vi "PPMS.TestLauncher.vi"() -> ()   [LabVIEW 2019, in "instrument.PPMS.lvclass"]
uses:
  instrument.PPMS.lvclass
  <vilib>/JKI/JKI SMO/SMO/SMO.lvclass
  <vilib>/JKI/JKI SMO/SMO/Typedefs/SMOState --Enum.ctl
  C:/Program Files (x86)/National Instruments/LabVIEW 2019/user.lib/LevyLab/Instrument Framework/Instrument Types/Cryostat/Instrument.Cryostat.lvclass
  C:/Program Files (x86)/National Instruments/LabVIEW 2019/user.lib/LevyLab/Instrument Framework/Instrument/Instrument.lvclass
  C:/Program Files (x86)/National Instruments/LabVIEW 2019/vi.lib/JKI/JKI SMO/SMO/SMO.lvclass
  <userlib>/LevyLab/Instrument Framework/Instrument/Instrument.lvclass
panel:
  in  "Debug Mode? [F]":bool
  out "SMO State":T1
  out "error out":errorcluster
  in  "Stop":bool
  # "PPMS Test Launcher"
  # "For instructions on how to use the JKI State Machine Objects, examples and video tutorials, visit:\nhttp://jki.net/state-machine-objects/\n\nJKI State Machine Objects™\nhttp://jki.net/state-machine-objects/\nCopyright (C) 2005-2015, JKI <info@jki.net>\nALL RIGHTS RESERVED"
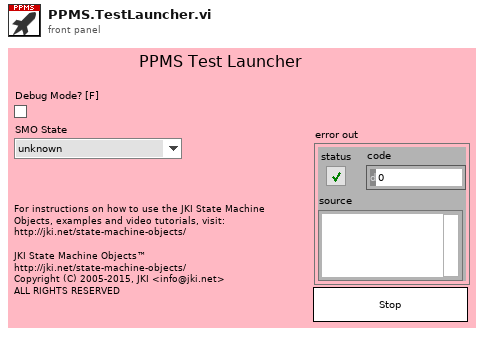
[diagram p1: front panel]
types:
  T1 = typedef "smo.lvlib/SMO.lvclass/SMOState --Enum.ctl" = enum16{"unknown", "Created", "Started", "Stopped"}
  T2 = typedef "smo.lvlib/SMO.lvclass/Public Events.ctl" = cluster{"Error":refnum<user-event>, "State":refnum<user-event>, "Reserve State":refnum<user-event>}
  T3 = cluster{"Event Registration Refnum":refnum<event-registration>}
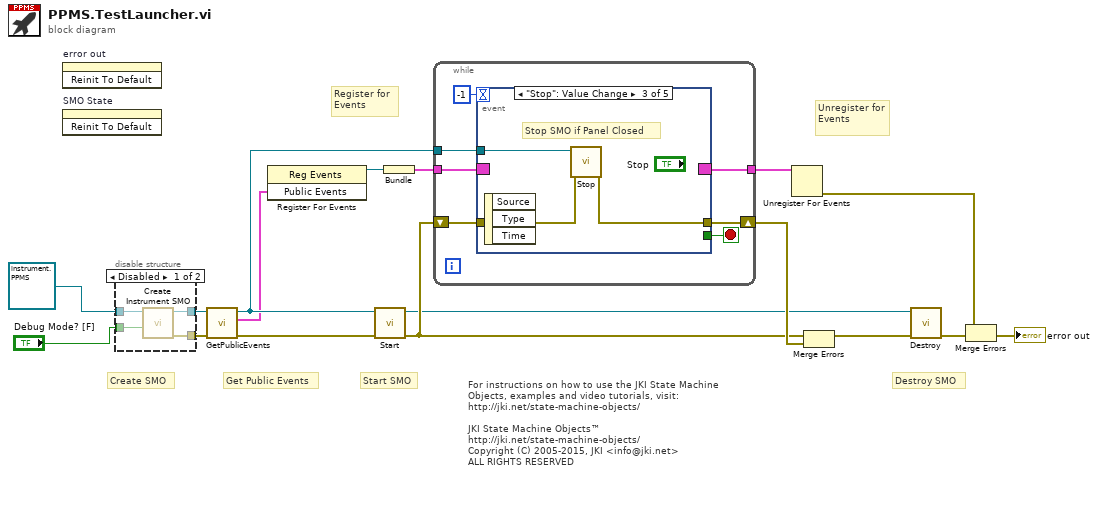
[diagram p0: block diagram]
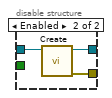
[diagram p2: hidden frame]
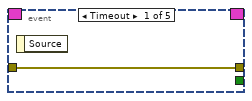
[diagram p3: hidden frame]
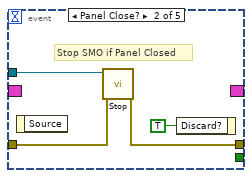
[diagram p4: hidden frame]
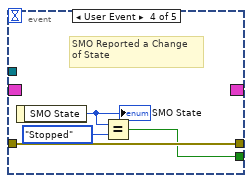
[diagram p5: hidden frame]
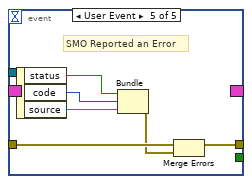
[diagram p6: hidden frame]
diagram:
  # "For instructions on how to use the JKI State Machine Objects, examples and video tutorials, visit:\nhttp://jki.net/state-machine-objects/\n\nJKI State Machine Objects™\nhttp://jki.net/state-machine-objects/\nCopyright (C) 2005-2015, JKI <info@jki.net>\nALL RIGHTS RESERVED"
  # "Get Public Events"
  # "Start SMO"
  # "Destroy SMO"
  # "Create SMO"
  # "Unregister for Events"
  # "Register for Events"
  n1 = invoke on="error out" class="Clust (strict)" method="Reinit To Default"() -> ()  [unwired: 3 in, 3 out]
  n2 = invoke on="SMO State" class="Enum (strict)" method="Reinit To Default"() -> ()  [unwired: 3 in, 3 out]
  n3 = disable-structure shown="Disabled" {
    disable-tunnel: [w21 w22] -> w8
    disable-tunnel: "Debug Mode? [F]" -> [w20 _]
    disable-tunnel: refnum<class "instrument.PPMS.lvclass"> refnum ("SMO.Template.lvclass") -> [w19 w24]
    disable-tunnel: [w18 w23] -> w1
    frame Disabled {
      n4 = call <userlib>:"Create Instrument SMO.vi"("Debug Mode? [F]"=w20, "Instrument in"=w19) -> ("error out"=w21:errorcluster, "Instrument out"=w18:refnum<class "instrument.PPMS.lvclass">)  [unwired: 8 in]
    }
    frame Enabled {
      n5 = call <vilib>:"Create.vi"("SMO"=w24) -> ("error out"=w22:errorcluster, "SMO out"=w23:refnum<class "instrument.PPMS.lvclass">)  [unwired: 8 in, 1 out]
    }
  }
  n6 = call <vilib>:"GetPublicEvents.vi"("error in (no error)"=w8, "SMO"=w1) -> ("error out"=w7:errorcluster, "Public Events"=w5:T2, "SMO out"=w6:refnum<class "instrument.PPMS.lvclass">)  [unwired: 7 in]
  n7 = register-events(w5) -> (reference out=w4:refnum<event-registration>)  [unwired: 2 in, 1 out]
  n8 = call <vilib>:"Start.vi"("error in (no error)"=w7, "SMO"=w6) -> ("error out"=w11:errorcluster, "SMO out"=w9:refnum<class "instrument.PPMS.lvclass">)  [unwired: 8 in]
  n9 = Bundle("Event Registration Refnum"=w4) -> (w16:T3)  [unwired: 1 in]
  n10 = while {
    shift-right: [w30] -> w15
    shift-left: w11 -> [w29]
    tunnel: w16 -> [w28]
    tunnel: [w27] -> w17
    tunnel: w6 -> [w26]
    stop <- w31 stop-if-true
    n11 = event shown="[2] \"Stop\": Value Change" {
      selector: w28 -> [_ _ _ _ _]
      dyn-events: [_ _ _ _ _] -> w27
      timeout: -1 -> [_ _ _ _ _]
      tunnel: [_ _ _ w40 _] -> w31
      tunnel: w26 -> [_ w36 w39 _ _]
      tunnel: [w32 w35 w38 w43 w47] -> w30
      tunnel: w29 -> [w32 w34 w37 w43 w45]
      event Timeout {
        n12 = event-data() -> ()  [unwired: 1 in, 1 out]
      }
      event Panel Close? {
        # "Stop SMO if Panel Closed"
        n13 = event-data() -> ()  [unwired: 1 in, 1 out]
        n14 = call <vilib>:"Stop.vi"("error in (no error)"=w34, "SMO"=w36) -> ("error out"=w35:errorcluster)  [unwired: 8 in, 1 out]
        n15 = event-data("Discard?"=TRUE ("OK")) -> ()  [unwired: 1 in, 1 out]
      }
      event "Stop": Value Change {
        # "Stop SMO if Panel Closed"
        n16 = event-data() -> ()  [unwired: 1 in, 3 out]
        n17 = call <vilib>:"Stop.vi"("error in (no error)"=w37, "SMO"=w39) -> ("error out"=w38:errorcluster)  [unwired: 8 in, 1 out]
      }
      event User Event {
        # "SMO Reported a Change\nof State"
        n18 = event-data() -> ("SMO State"=w42:T1)  [unwired: 1 in]
        "SMO State" <- w42
        n19 = Equal?(x=w42, y=SMOState_--Enum."Stopped") -> (x = y?=w40:bool)
      }
      event User Event {
        # "SMO Reported an Error"
        n20 = event-data() -> ("status"=w46:bool, "code"=w49:i32, "source"=w48:string)  [unwired: 1 in]
        n21 = Bundle("status"=w46, "code"=w49, "source"=w48) -> (w44:errorcluster)  [unwired: 1 in]
        n22 = Merge Errors(w45, w44) -> (w47:errorcluster)
      }
    }
  }
  n23 = Unregister For Events(event registration refnum=w17) -> (error out=w14:errorcluster)  [unwired: 1 in]
  n24 = Merge Errors(w11, w15) -> (w10:errorcluster)
  n25 = call <vilib>:"Destroy.vi"("error in (no error)"=w10, "SMO"=w9) -> ("error out"=w12:errorcluster)  [unwired: 9 in]
  n26 = Merge Errors(w14, w12) -> (→"error out":errorcluster)
